vi "dvp Vi Is Valid.vi"(10 "pIsValid":i32, 11 "handle":u32) -> (2 "pIsValid out":i32, 3 "function return":u32(ring))   [LabVIEW 2018, in "LabViewDVPCamera.lvlib"]
doc: "LabviewDvp2Api dvpStatus dvpViIsValid(dvpHandle handle, BOOL *pIsValid);"
uses:
  LabViewDVPCamera.lvlib
  LabViewDVPCamera/LabViewDVPCamera.dll
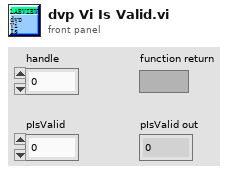
[diagram p1: front panel]
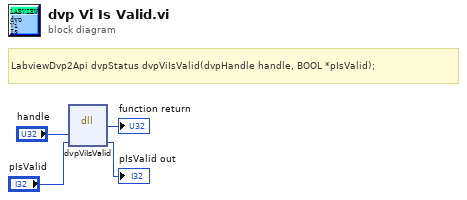
[diagram p0: block diagram]
diagram:
  # "LabviewDvp2Api dvpStatus dvpViIsValid(dvpHandle handle, BOOL *pIsValid);"
  n1 = dll-call lib="C:/Program Files (x86)/DVP2 Labview cn 64/Sample/LabViewDVPCamera/LabViewDVPCamera.*" fn="dvpViIsValid"("handle"="handle", "pIsValid"="pIsValid") -> (→"function return":u32, "pIsValid"=→"pIsValid out":i32)  [unwired: 4 in, 2 out]
